vi "NET_RIO_Status.vi"(8 "Read(F) Write(T)":bool, 11 "RoboRio Status In":T1) -> (3 "RoboRio Status Out":T1)   [LabVIEW 2017]
uses:
  _SHARE ALL/TypeDef Share All/CLUSTER_RoboRio_Status.ctl
  _SHARE ALL/TypeDef Share All/CLUSTER_RoboRio_Faults.ctl
  _SHARE ALL/TypeDef Share All/CLUSTER_RoboRio_Rails.ctl
  _SHARE ALL/TypeDef Share All/CLUSTER_RoboRio_SingleRail.ctl
  <vilib>/Rock Robotics/Network Tables/NT Write Numeric Array.vi
  <vilib>/Rock Robotics/Network Tables/NT Write Boolean Array.vi
  <vilib>/Rock Robotics/Network Tables/NT Read Numeric Array.vi
  <vilib>/Rock Robotics/Network Tables/NT Read Boolean Array.vi
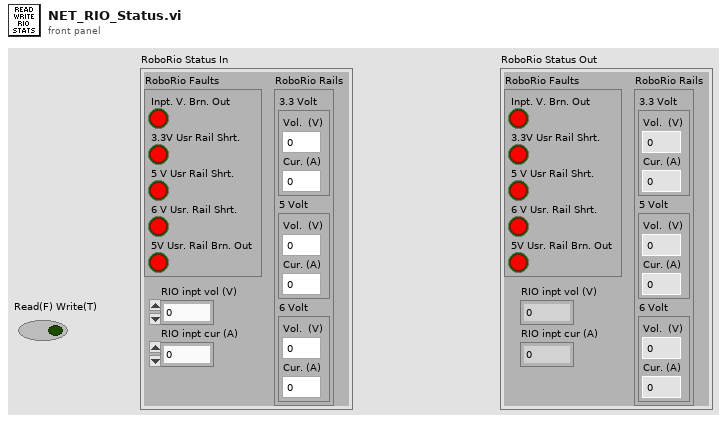
[diagram p1: front panel]
types:
  T1 = typedef "CLUSTER_RoboRio_Status.ctl" = cluster{"RoboRio Faults":T2, "RIO inpt vol (V)":dbl, "RIO inpt cur (A)":dbl, "RoboRio Rails":T3}
  T2 = typedef "CLUSTER_RoboRio_Faults.ctl" = cluster{"Inpt. V. Brn. Out":bool, "3.3V Usr Rail Shrt.":bool, "5 V Usr Rail Shrt.":bool, "6 V Usr. Rail Shrt.":bool, "5V Usr. Rail Brn. Out":bool}
  T3 = typedef "CLUSTER_RoboRio_Rails.ctl" = cluster{"3.3 Volt":T4, "5 Volt":T4, "6 Volt":T4}
  T4 = typedef "CLUSTER_RoboRio_SingleRail.ctl" = cluster{"Vol.  (V)":dbl, "Cur. (A)":dbl}
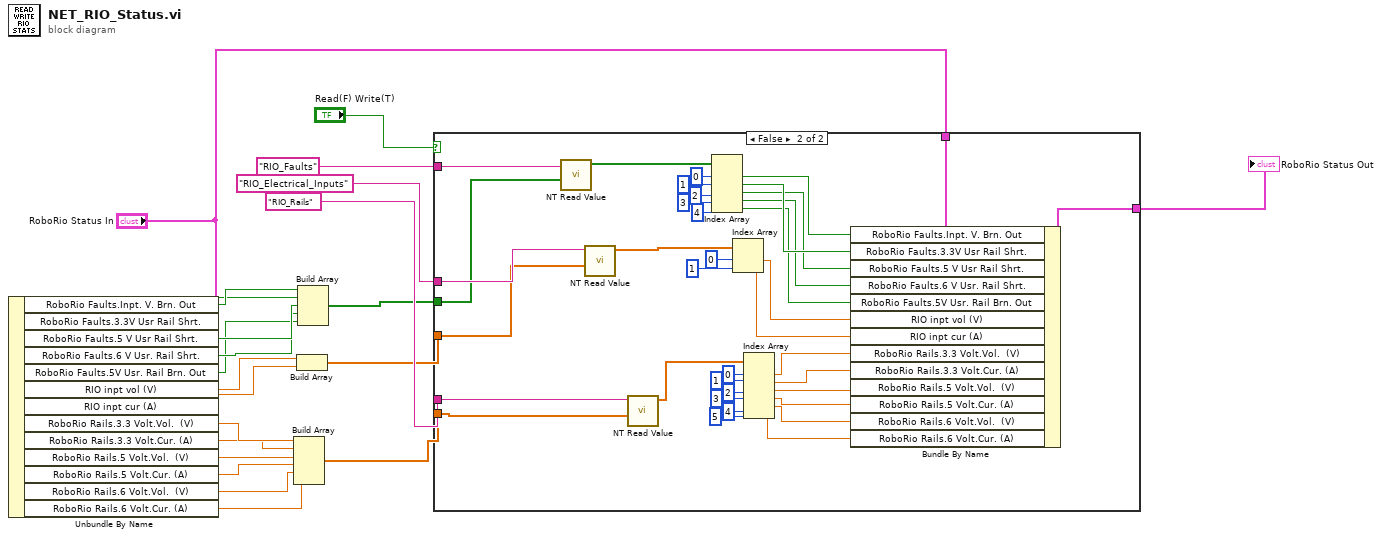
[diagram p0: block diagram]
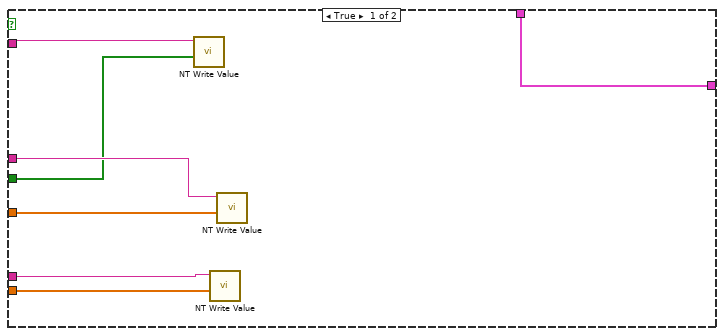
[diagram p2: hidden frame]
diagram:
  n1 = Unbundle By Name("RoboRio Status In") -> ("RoboRio Faults.Inpt. V. Brn. Out"=w5:bool, "RoboRio Faults.3.3V Usr Rail Shrt."=w4:bool, "RoboRio Faults.5 V Usr Rail Shrt."=w3:bool, "RoboRio Faults.6 V Usr. Rail Shrt."=w2:bool, "RoboRio Faults.5V Usr. Rail Brn. Out"=w1:bool, "RIO inpt vol (V)"=w16:dbl, "RIO inpt cur (A)"=w15:dbl, "RoboRio Rails.3.3 Volt.Vol.  (V)"=w12:dbl, "RoboRio Rails.3.3 Volt.Cur. (A)"=w11:dbl, "RoboRio Rails.5 Volt.Vol.  (V)"=w10:dbl, "RoboRio Rails.5 Volt.Cur. (A)"=w9:dbl, "RoboRio Rails.6 Volt.Vol.  (V)"=w8:dbl, "RoboRio Rails.6 Volt.Cur. (A)"=w7:dbl)
  n2 = Build Array(w12, w11, w10, w9, w8, w7) -> (w6:dbl[])
  n3 = Build Array(w16, w15) -> (w14:dbl[])
  n4 = Build Array(w5, w4, w3, w2, w1) -> (w13:bool[])
  n5 = case shown="False" "Read(F) Write(T)" {
    tunnel: "RIO_Faults" ("Name") -> [w29 w66]
    tunnel: [w23 w30] -> w17
    tunnel: "RIO_Electrical_Inputs" ("Name") -> [w28 w65]
    tunnel: "RIO_Rails" ("Name") -> [w25 w64]
    tunnel: "RoboRio Status In" -> [w23 w31]
    tunnel: w13 -> [w27 w63]
    tunnel: w14 -> [w26 w62]
    tunnel: w6 -> [w24 w47]
    frame True {
      n6 = call-poly <vilib>:"NT Write Value.vi"("Boolean Array"=w27, "Name"=w29) -> ()  [unwired: 9 in, 1 out]
      n7 = call-poly <vilib>:"NT Write Value.vi"("Numeric Array"=w24, "Name"=w25) -> ()  [unwired: 9 in, 1 out]
      n8 = call-poly <vilib>:"NT Write Value.vi"("Numeric Array"=w26, "Name"=w28) -> ()  [unwired: 9 in, 1 out]
    }
    frame False {
      n9 = call-poly <vilib>:"NT Read Value.vi"("Default Value"=w63, "Name"=w66) -> ("Boolean Array"=w58:bool[])  [unwired: 8 in, 1 out]
      n10 = call-poly <vilib>:"NT Read Value.vi"("Default Value"=w62, "Name"=w65) -> ("Numeric Array"=w61:dbl[])  [unwired: 8 in, 1 out]
      n11 = call-poly <vilib>:"NT Read Value.vi"("Default Value"=w47, "Name"=w64) -> ("Numeric Array"=w44:dbl[])  [unwired: 8 in, 1 out]
      n12 = Index Array(array=w58, index #1=0 ("index"), index #2=1 ("index"), index #3=2 ("index"), index #4=3 ("index"), index #5=4 ("index")) -> (element #1=w57:bool, element #2=w56:bool, element #3=w55:bool, element #4=w54:bool, element #5=w53:bool)
      n13 = Index Array(array=w61, index #1=0 ("index"), index #2=1 ("index")) -> (element #1=w46:dbl, element #2=w45:dbl)
      n14 = Index Array(array=w44, index #1=0 ("index"), index #2=1 ("index"), index #3=2 ("index"), index #4=3 ("index"), index #5=4 ("index"), index #6=5 ("index")) -> (element #1=w37:dbl, element #2=w36:dbl, element #3=w35:dbl, element #4=w34:dbl, element #5=w33:dbl, element #6=w32:dbl)
      n15 = Bundle By Name(cluster=w31, "RoboRio Faults.Inpt. V. Brn. Out"=w57, "RoboRio Faults.3.3V Usr Rail Shrt."=w56, "RoboRio Faults.5 V Usr Rail Shrt."=w55, "RoboRio Faults.6 V Usr. Rail Shrt."=w54, "RoboRio Faults.5V Usr. Rail Brn. Out"=w53, "RIO inpt vol (V)"=w46, "RIO inpt cur (A)"=w45, "RoboRio Rails.3.3 Volt.Vol.  (V)"=w37, "RoboRio Rails.3.3 Volt.Cur. (A)"=w36, "RoboRio Rails.5 Volt.Vol.  (V)"=w35, "RoboRio Rails.5 Volt.Cur. (A)"=w34, "RoboRio Rails.6 Volt.Vol.  (V)"=w33, "RoboRio Rails.6 Volt.Cur. (A)"=w32) -> (w30:T1)
    }
  }
  "RoboRio Status Out" <- w17
